vi "Conf Resistance.vi"(0 "VISA Resource Name":refnum<visa-resource-name>, 1 "Check/Set (F:Set)":bool, 2 "Check Parameter (1:Ap Min)":T3(ring)=enum."Aperture Min", 5 "4 Wire/2 Wire (F:2)":bool, 7 "Autorange? (F:OFF)":bool, 9 "Range (8:Maximum)":T2(ring)=enum."Maximum", 11 "error in (no error)":errorcluster, 12 "Channel List (empty)":string, 13 "Advanced Config":T1={"Offset Compensation (F:Off)"=FALSE, "Aperture Value (.4)"=0.4, "Aperture (1:Minimum)"=1, "NPLC (1)"=2, "Integration Time (F:Aperture)"=FALSE} {"NPLC (1)" items=[".02", ".2", "1", "2", "10", "20", "100", "200", "Minimum", "Maximum"]; "Aperture (1:Minimum)" items=["Manual", "Minimum", "Maximum"]; "Aperture Value (.4)" min=0.4 max=4.0 format="%.2f"}) -> (4 "VISA Resource Name Out":refnum<visa-resource-name>, 8 "Configuration?":string, 15 "error out":errorcluster)   [LabVIEW 2016, in "Agilent 34970.lvlib"]
doc: "This VI configures the instrument for advanced resistance measurements.\n\nThis is an advanced measurment configuration VI. For more information on the different ways to take and configure a measurment, refer to the context help and block diagram of \"HP34970A Advanced Scan Example.vi\"."
uses:
  Agilent 34970.lvlib
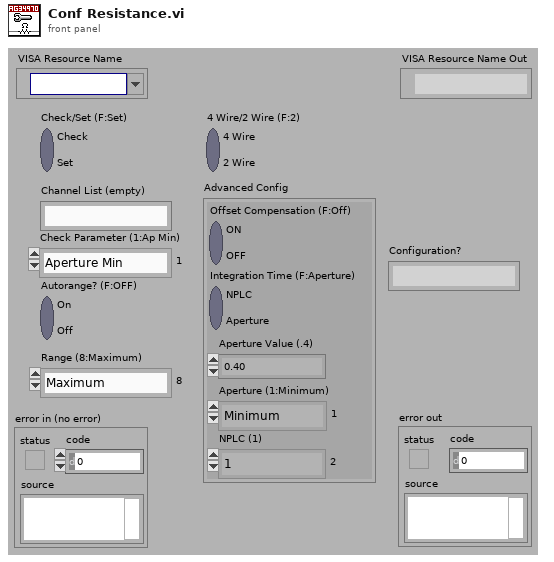
[diagram p1: front panel]
types:
  T1 = cluster{"Offset Compensation (F:Off)":bool, "Aperture Value (.4)":dbl, "Aperture (1:Minimum)":u16, "NPLC (1)":u16, "Integration Time (F:Aperture)":bool}
  T2 = enum16{"100 Ohm", "1 kOhm", "10 kOhm", "100 kOhm", "1 MOhm", "10 MOhm", "100 MOhm", "Minimum", "Maximum"}
  T3 = enum16{"Aperture (By Chan)", "Aperture Min", "Aperture Max", "NPLC (By Chan)", "NPLC Min", "NPLC Max", "2-Wire Offset Comp", "4-Wire Offset Comp"}
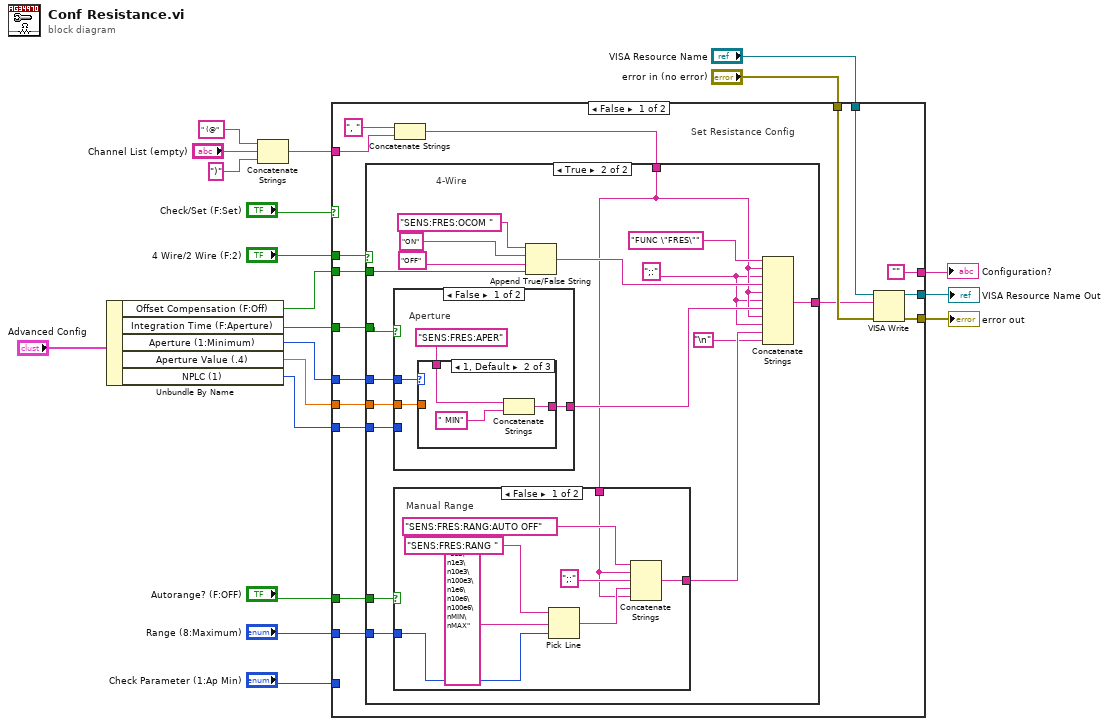
[diagram p0: block diagram]
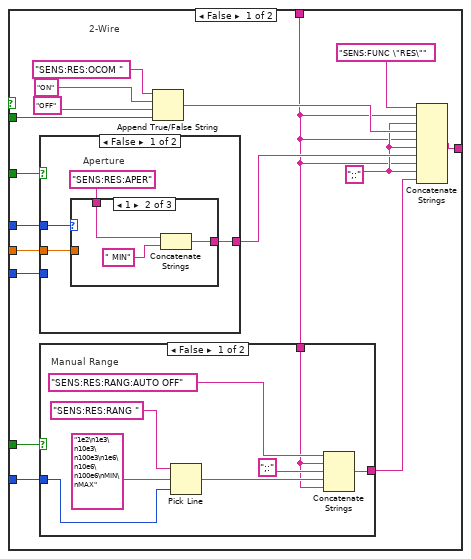
[diagram p2: hidden frame]
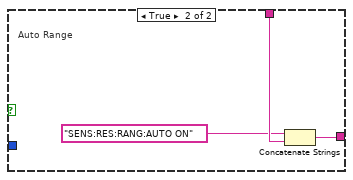
[diagram p3: hidden frame]
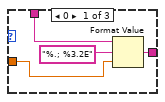
[diagram p4: hidden frame]
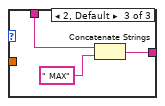
[diagram p5: hidden frame]
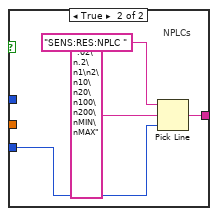
[diagram p6: hidden frame]
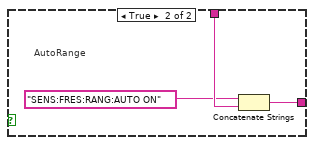
[diagram p7: hidden frame]
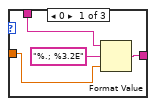
[diagram p8: hidden frame]
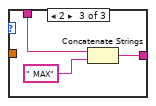
[diagram p9: hidden frame]
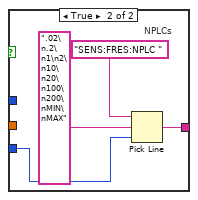
[diagram p10: hidden frame]
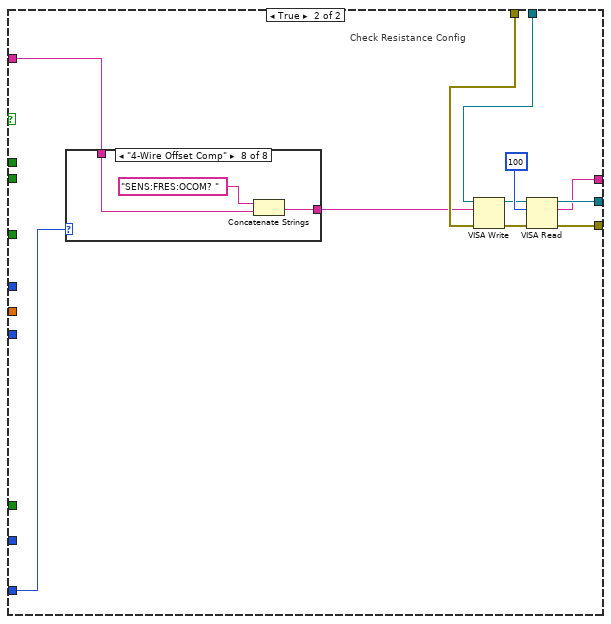
[diagram p11: hidden frame]
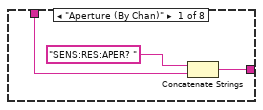
[diagram p12: hidden frame]
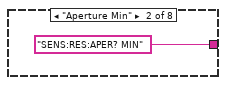
[diagram p13: hidden frame]
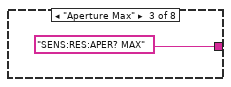
[diagram p14: hidden frame]
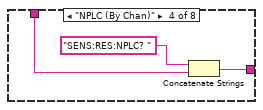
[diagram p15: hidden frame]
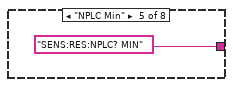
[diagram p16: hidden frame]
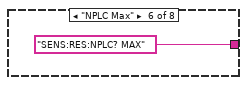
[diagram p17: hidden frame]
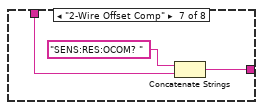
[diagram p18: hidden frame]
diagram:
  n1 = Unbundle By Name("Advanced Config") -> ("Offset Compensation (F:Off)"=w12:bool, "Integration Time (F:Aperture)"=w11:bool, "Aperture (1:Minimum)"=w10:u16, "Aperture Value (.4)"=w9:dbl, "NPLC (1)"=w8:u16)
  n2 = Concatenate Strings(" (@", "Channel List (empty)", ")") -> (w15:string)
  n3 = case shown="False" "Check/Set (F:Set)" {
    tunnel: [w34 w141] -> w4
    tunnel: [w35 w139] -> w5
    tunnel: "4 Wire/2 Wire (F:2)" -> [w33 _]
    tunnel: w15 -> [w30 w133]
    tunnel: ["" ("Empty String Constant") w132] -> w14
    tunnel: "VISA Resource Name" -> [w37 w135]
    tunnel: "error in (no error)" -> [w36 w136]
    tunnel: w12 -> [w31 _]
    tunnel: w11 -> [w28 _]
    tunnel: w10 -> [w27 _]
    tunnel: w9 -> [w26 _]
    tunnel: w8 -> [w25 _]
    tunnel: "Check Parameter (1:Ap Min)" -> [_ w134]
    tunnel: "Range (8:Maximum)" -> [w23 _]
    tunnel: "Autorange? (F:OFF)" -> [w22 _]
    frame False {
      # "Set Resistance Config"
      n4 = Concatenate Strings(", ", w30) -> (w32:string)
      n5 = case shown="True" w33 {
        tunnel: w32 -> [w38 w88]
        tunnel: w31 -> [w54 w99]
        tunnel: w28 -> [w48 w92]
        tunnel: w27 -> [w47 w96]
        tunnel: w26 -> [w46 w97]
        tunnel: w25 -> [w45 w98]
        tunnel: [w43 w91] -> w21
        tunnel: w23 -> [w42 w89]
        tunnel: w22 -> [w41 w90]
        frame False {
          w40 = ";:"
          # "2-Wire"
          n6 = case shown="False" w48 {
            tunnel: w46 -> [w68 _]
            tunnel: w47 -> [w67 _]
            tunnel: w45 -> [_ w80]
            tunnel: [w66 w81] -> w44
            frame False {
              # "Aperture"
              n7 = case shown="1" w67 {
                tunnel: "SENS:RES:APER" -> [w73 w76 w78]
                tunnel: [w71 w74 w77] -> w66
                tunnel: w68 -> [w70 _ _]
                frame 0 {
                  n8 = Format Value(string ("")=w73, format string="%.; %3.2E", value (0)=w70) -> (output string=w71:string)
                }
                frame 1 {
                  n9 = Concatenate Strings(w76, " MIN") -> (w74:string)
                }
                frame 2, Default {
                  n10 = Concatenate Strings(w78, " MAX") -> (w77:string)
                }
              }
            }
            frame True {
              # "NPLCs"
              n11 = Pick Line(string ("")="SENS:RES:NPLC ", multi-line string=".02\n.2\n1\n2\n10\n20\n100\n200\nMIN\nMAX", line index=w80) -> (output string=w81:string)
            }
          }
          n12 = case shown="False" w41 {
            tunnel: w42 -> [w60 _]
            tunnel: w38 -> [w56 w65]
            tunnel: [w55 w63] -> w39
            frame False {
              # "Manual Range"
              n13 = Pick Line(string ("")="SENS:RES:RANG ", multi-line string="1e2\n1e3\n10e3\n100e3\n1e6\n10e6\n100e6\nMIN\nMAX", line index=w60) -> (output string=w57:string)
              n14 = Concatenate Strings("SENS:RES:RANG:AUTO OFF", w56, ";:", w57, w56) -> (w55:string)
            }
            frame True {
              # "Auto Range"
              n15 = Concatenate Strings("SENS:RES:RANG:AUTO ON", w65) -> (w63:string)
            }
          }
          n16 = Append True/False String(1:w54, 2:"OFF" ("false string"), 3:"ON" ("true string"), 4:"SENS:RES:OCOM ") -> (0:w49:string)
          n17 = Concatenate Strings("SENS:FUNC \"RES\"", w38, w40, w49, w38, w40, w44, w38, w40, w39) -> (w43:string)
        }
        frame True {
          w87 = ";:"
          # "4-Wire"
          n18 = case shown="False" w92 {
            tunnel: w97 -> [w115 _]
            tunnel: w96 -> [w114 _]
            tunnel: w98 -> [_ w128]
            tunnel: [w113 w127] -> w93
            frame False {
              # "Aperture"
              n19 = case shown="1, Default" w114 {
                tunnel: "SENS:FRES:APER" -> [w120 w123 w125]
                tunnel: [w118 w121 w124] -> w113
                tunnel: w115 -> [w117 _ _]
                frame 0 {
                  n20 = Format Value(string ("")=w120, format string="%.; %3.2E", value (0)=w117) -> (output string=w118:string)
                }
                frame 1, Default {
                  n21 = Concatenate Strings(w123, " MIN") -> (w121:string)
                }
                frame 2 {
                  n22 = Concatenate Strings(w125, " MAX") -> (w124:string)
                }
              }
            }
            frame True {
              # "NPLCs"
              n23 = Pick Line(string ("")="SENS:FRES:NPLC ", multi-line string=".02\n.2\n1\n2\n10\n20\n100\n200\nMIN\nMAX", line index=w128) -> (output string=w127:string)
            }
          }
          n24 = case shown="False" w90 {
            tunnel: w89 -> [w102 _]
            tunnel: w88 -> [w104 w112]
            tunnel: [w103 w110] -> w86
            frame False {
              # "Manual Range"
              n25 = Pick Line(string ("")="SENS:FRES:RANG ", multi-line string="1e2\n1e3\n10e3\n100e3\n1e6\n10e6\n100e6\nMIN\nMAX", line index=w102) -> (output string=w105:string)
              n26 = Concatenate Strings("SENS:FRES:RANG:AUTO OFF", w104, ";:", w105, w104) -> (w103:string)
            }
            frame True {
              # "AutoRange"
              n27 = Concatenate Strings("SENS:FRES:RANG:AUTO ON", w112) -> (w110:string)
            }
          }
          n28 = Append True/False String(1:w99, 2:"OFF" ("false string"), 3:"ON" ("true string"), 4:"SENS:FRES:OCOM ") -> (0:w94:string)
          n29 = Concatenate Strings("FUNC \"FRES\"", w88, w87, w94, w88, w87, w93, w88, w87, w86, "\n" ("Line Feed Constant")) -> (w91:string)
        }
      }
      n30 = VISA Write(VISA resource name=w37, write buffer=w21, error in (no error)=w36) -> (VISA resource name out=w35:refnum<visa-resource-name>, error out=w34:errorcluster)  [unwired: 1 out]
    }
    frame True {
      # "Check Resistance Config"
      n31 = case shown="\"4-Wire Offset Comp\"" w134 {
        tunnel: [w143 "SENS:RES:APER? MIN" "SENS:RES:APER? MAX" w148 "SENS:RES:NPLC? MIN" "SENS:RES:NPLC? MAX" w153 w155] -> w131
        tunnel: w133 -> [w142 _ _ w147 _ _ w152 w156]
        frame "Aperture (By Chan)" {
          n32 = Concatenate Strings("SENS:RES:APER? ", w142) -> (w143:string)
        }
        frame "Aperture Min" {
        }
        frame "Aperture Max" {
        }
        frame "NPLC (By Chan)" {
          n33 = Concatenate Strings("SENS:RES:NPLC? ", w147) -> (w148:string)
        }
        frame "NPLC Min" {
        }
        frame "NPLC Max" {
        }
        frame "2-Wire Offset Comp" {
          n34 = Concatenate Strings("SENS:RES:OCOM? ", w152) -> (w153:string)
        }
        frame "4-Wire Offset Comp" {
          n35 = Concatenate Strings("SENS:FRES:OCOM? ", w156) -> (w155:string)
        }
      }
      n36 = VISA Write(VISA resource name=w135, write buffer=w131, error in (no error)=w136) -> (VISA resource name out=w138:refnum<visa-resource-name>, error out=w137:errorcluster)  [unwired: 1 out]
      n37 = VISA Read(VISA resource name=w138, byte count=u32 100 ("byte count (0)"), error in (no error)=w137) -> (VISA resource name out=w139:refnum<visa-resource-name>, read buffer=w132:string, error out=w141:errorcluster)  [unwired: 1 out]
    }
  }
  "Configuration?" <- w14
  "error out" <- w4
  "VISA Resource Name Out" <- w5
